vi "Symphony MultiAccu_Config.vi"(6 "MultiAcqHardwareMode":bool, 7 "Cleans Before":i32=1, 8 "error in (no error)":errorcluster, 9 "MultiAcqShutterMode":i32(ring)=1 items=["jyMultiAcqStateBeforeFirstOnly"=1, "jyMultiAcqStateBeforeEach"=3], 10 "Accumulations:":u16=1 min=1 step=1, 11 "JYCCDLib.IJYCCDReqd":refnum<k7>) -> (0 "error out":errorcluster, 3 "JYCCDLib.IJYCCDReqd":refnum<k7>)   [LabVIEW 2012]
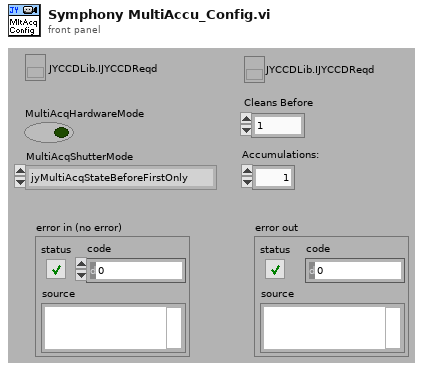
[diagram p1: front panel]
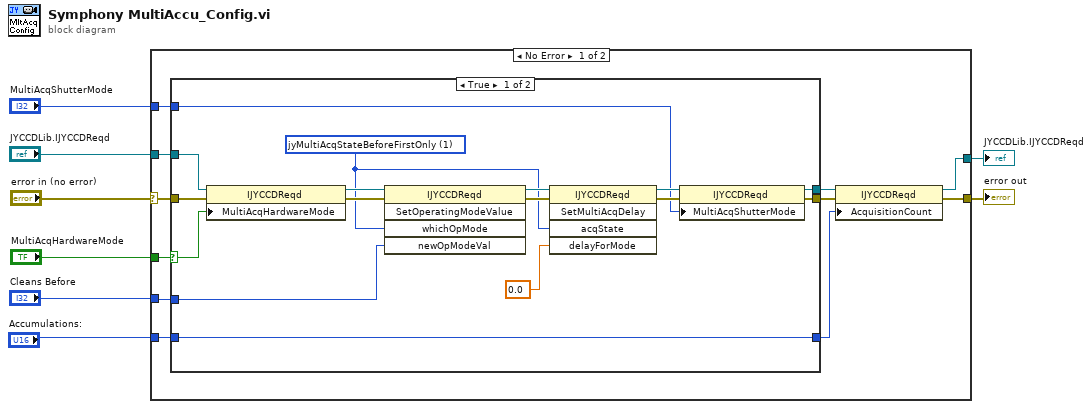
[diagram p0: block diagram]
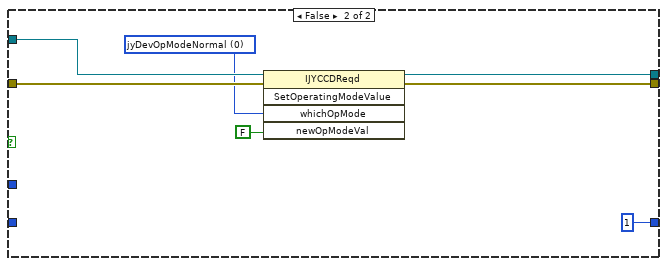
[diagram p2: hidden frame]
diagram:
  n1 = case shown="No Error" "error in (no error)" {
    selector: "error in (no error)" -> [w15 w44]
    tunnel: "Accumulations:" -> [w10 _]
    tunnel: "JYCCDLib.IJYCCDReqd" -> [w17 w43]
    tunnel: "MultiAcqHardwareMode" -> [w9 _]
    tunnel: "Cleans Before" -> [w16 _]
    tunnel: "MultiAcqShutterMode" -> [w14 _]
    tunnel: [w13 w44] -> w3
    tunnel: [w12 w43] -> w2
    frame No Error {
      n2 = case shown="True" w9 {
        selector: w9 -> [w21 _]
        tunnel: [w30 w37] -> w19
        tunnel: [w29 w38] -> w18
        tunnel: w17 -> [w28 w40]
        tunnel: w16 -> [w25 _]
        tunnel: w15 -> [w20 w41]
        tunnel: w14 -> [w24 _]
        tunnel: [w22 u16 1 ("Accumulations:")] -> w11
        tunnel: w10 -> [w22 _]
        frame True {
          w23 = 1 items=["jyMultiAcqStateNever", "jyMultiAcqStateBeforeFirstOnly", "jyMultiAcqStateBetweenOnly", "jyMultiAcqStateBeforeEach"] ("acqState")
          n3 = property class="IJYCCDReqd"(reference=w28, error in=w20, "MultiAcqHardwareMode"=w21) -> (reference out=w27:refnum<k7>, error out=w26:errorcluster)
          n4 = invoke class="IJYCCDReqd" method="SetOperatingModeValue"(reference=w27, error in=w26, "whichOpMode"=w23, "newOpModeVal"=w25) -> (reference out=w35:refnum<k7>, error out=w34:errorcluster)  [unwired: 1 in, 3 out]
          n5 = invoke class="IJYCCDReqd" method="SetMultiAcqDelay"(reference=w35, error in=w34, "acqState"=w23, "delayForMode"=0.0) -> (reference out=w32:refnum<k7>, error out=w31:errorcluster)  [unwired: 1 in, 3 out]
          n6 = property class="IJYCCDReqd"(reference=w32, error in=w31, "MultiAcqShutterMode"=w24) -> (reference out=w30:refnum<k7>, error out=w29:errorcluster)
        }
        frame False {
          w39 = 0 items=["jyDevOpModeNormal", "jyDevOpModeAcqHWTimeBased", "jyDevOpModeAcqSWTimeBased", "jyDevOpModeAcqFKBurst", "jyDevOpModeAcqFKBlast", "jyDevOpModeAcqICCD", "jyDevOpModeAcqAllowIntermediateRead", "jyDevOpModeLAST"] ("whichOpMode")
          n7 = invoke class="IJYCCDReqd" method="SetOperatingModeValue"(reference=w40, error in=w41, "whichOpMode"=w39, "newOpModeVal"=FALSE) -> (reference out=w37:refnum<k7>, error out=w38:errorcluster)  [unwired: 1 in, 3 out]
        }
      }
      n8 = property class="IJYCCDReqd"(reference=w19, error in=w18, "AcquisitionCount"=w11) -> (reference out=w12:refnum<k7>, error out=w13:errorcluster)
    }
    frame Error {
    }
  }
  "JYCCDLib.IJYCCDReqd" <- w2
  "error out" <- w3
